vi "programa 5.vi"() -> ()   [LabVIEW 2011]
panel:
  out "Personas":dbl
  in  "Planta":u16(ring) items=["Planta #1", "Planta #2", "Planta #3"]
  out "A/c":bool
  out "Temperatura":i32(slide) scale=0.0..60.0
  # "Se genera la temperatura entre 1-60,\nse selecciona la planta usando el menu ring,\nluego se gnera el numero de personas entre 1-50"
  # "planta 1 si hay mas de 25 personas y la temperatura\nes mayor a 22 se enciende el A/C\n\nplanta 2 si hay mas de 30 personas y la temperatura\nes mayor a 27 se enciende el A/C\n\nplanta 3 si hay mas de 20 personas y la temperatura\nes mayor a 29 se enciende el A/C"
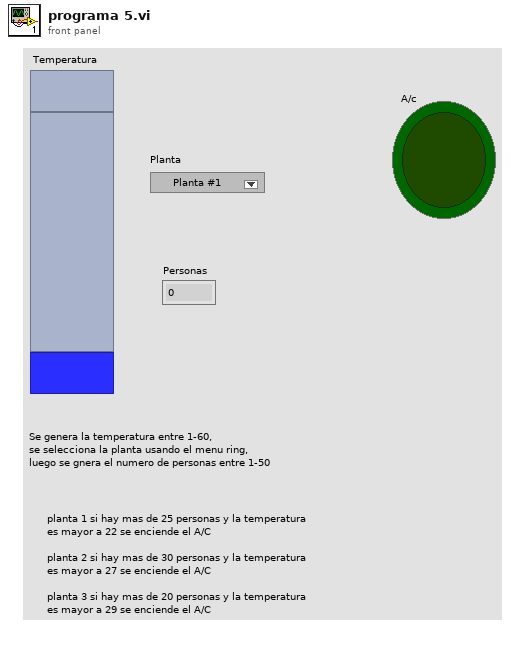
[diagram p1: front panel]
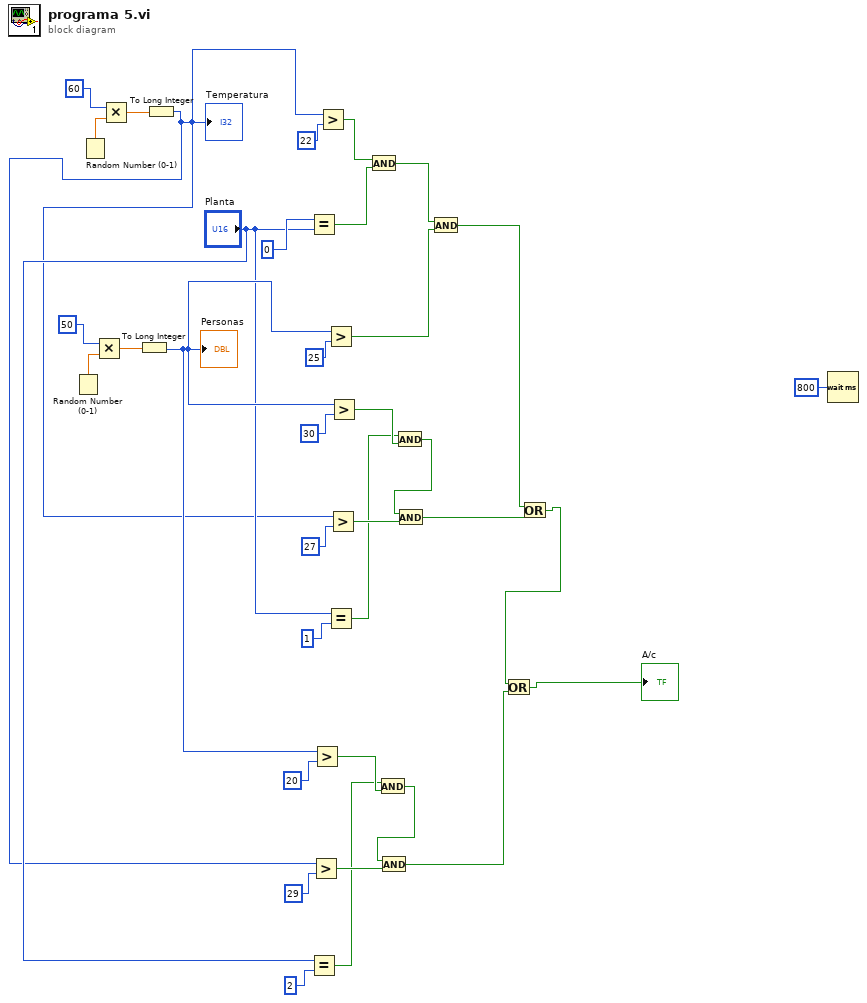
[diagram p0: block diagram]
diagram:
  n1 = Random Number (0-1)() -> (number: 0 to 1=w32:dbl)
  n2 = Random Number (0-1)() -> (number: 0 to 1=w35:dbl)
  n3 = Multiply(x=50, y=w32) -> (x*y=w31:dbl)
  n4 = Multiply(x=60, y=w35) -> (x*y=w34:dbl)
  n5 = To Long Integer(number=w31) -> (32bit integer=w9:i32)
  "Personas" <- w9
  n6 = To Long Integer(number=w34) -> (32bit integer=w7:i32)
  "Temperatura" <- w7
  n7 = Equal?(x=0, y="Planta") -> (x = y?=w25:bool)
  n8 = Equal?(x="Planta", y=u16 2) -> (x = y?=w10:bool)
  n9 = Greater?(x=w7, y=29) -> (0:w12:bool)
  n10 = Greater?(x=w9, y=20) -> (0:w13:bool)
  n11 = Greater?(x=w7, y=22) -> (0:w28:bool)
  n12 = Greater?(x=w9, y=25) -> (0:w24:bool)
  n13 = Equal?(x="Planta", y=u16 1) -> (x = y?=w17:bool)
  n14 = Greater?(x=w7, y=27) -> (0:w19:bool)
  n15 = Greater?(x=w9, y=30) -> (0:w20:bool)
  n16 = And(x=w28, y=w25) -> (x .and. y?=w26:bool)
  n17 = And(x=w10, y=w13) -> (x .and. y?=w11:bool)
  n18 = And(x=w11, y=w12) -> (x .and. y?=w3:bool)
  n19 = And(x=w17, y=w20) -> (x .and. y?=w18:bool)
  n20 = And(x=w18, y=w19) -> (x .and. y?=w5:bool)
  n21 = And(x=w26, y=w24) -> (x .and. y?=w6:bool)
  n22 = Or(x=w6, y=w5) -> (x .or. y?=w4:bool)
  n23 = Or(x=w4, y=w3) -> (x .or. y?=→"A/c":bool)
  n24 = Wait (ms)(milliseconds to wait=u32 800) -> ()  [unwired: 1 out]
